vi "Get SmartCard Variable Names.vi"(8 "error in":errorcluster, 11 "Dataset Name":string) -> (0 "error out":errorcluster, 3 "Variable Names":string[](array[string]))   [LabVIEW 2015, in "Support VIs.lvlib"]
uses:
  QMH_Topside/Support VIs/Support VIs.lvlib
panel:
  out "name":string
  out "text":string
  out "stripped path":path
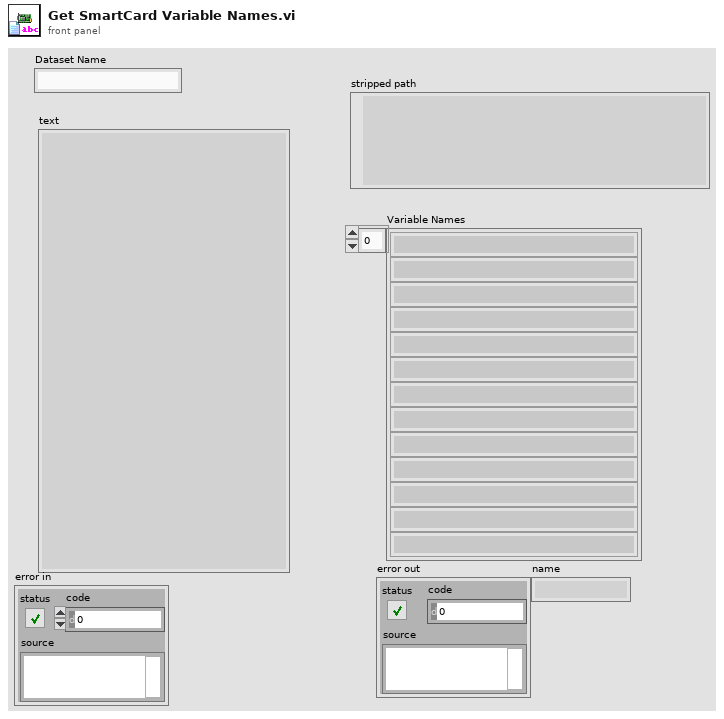
[diagram p1: front panel]
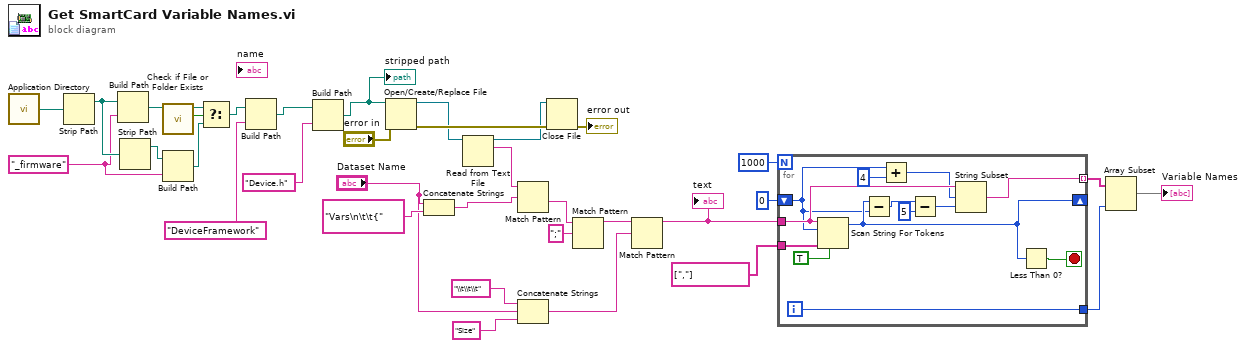
[diagram p0: block diagram]
diagram:
  w2 = "_firmware" ("name or relative path")
  n1 = call <vilib>:"Application Directory.vi"() -> ("Application Directory"=w35:path)
  n2 = Strip Path(path=w35) -> (stripped path=w4:path)  [unwired: 1 out]
  n3 = Build Path(base path=w4, name or relative path=w2) -> (appended path=w5:path)
  n4 = Strip Path(path=w4) -> (stripped path=w3:path)  [unwired: 1 out]
  n5 = call <vilib>:"Check if File or Folder Exists.vi"("path"=w5) -> ("file or folder exists?"=w8:bool, "dup path"=w7:path)  [unwired: 8 in, 1 out]
  n6 = Build Path(base path=w3, name or relative path=w2) -> (appended path=w1:path)
  n7 = Select(t=w7, s=w8, f=w1) -> (s? t:f=w6:path)
  n8 = Build Path(base path=w6, name or relative path="DeviceFramework") -> (appended path=w11:path)
  n9 = Build Path(base path=w11, name or relative path="Device.h") -> (appended path=w33:path)
  "stripped path" <- w33
  n10 = Open/Create/Replace File(file path (use dialog)=w33, error in="error in") -> (refnum out=w31:refnum<file>, error out=w32:errorcluster)  [unwired: 4 in, 1 out]
  n11 = Concatenate Strings("Dataset Name", "Vars\n\t\t{" ("regular expression")) -> (w20:string)
  n12 = Read from Text File(file (use dialog)=w31) -> (refnum out=w30:refnum<file>, text=w29:string)  [unwired: 3 in, 2 out]
  n13 = Match Pattern(string=w29, regular expression=w20) -> (after substring=w28:string)  [unwired: 1 in, 3 out]
  n14 = Concatenate Strings("\\t\\t\\t" ("string"), "Dataset Name", "Size" ("string")) -> (w16:string)
  n15 = Close File(refnum=w30, error in=w32) -> (error out=→"error out":errorcluster)  [unwired: 1 out]
  n16 = Match Pattern(string=w28, regular expression=";") -> (before substring=w25:string)  [unwired: 1 in, 3 out]
  n17 = Match Pattern(string=w25, regular expression=w16) -> (before substring=w24:string)  [unwired: 1 in, 3 out]
  "text" <- w24
  n18 = for {
    N: 1000 -> [_]
    tunnel: string[] [","] ("delimiters (\\s,\\t,\\r,\\n)") -> [w48]
    shift-right: [w41] -> _
    shift-left: 0 ("offset past token") -> [w40]
    tunnel: w24 -> [w45]
    tunnel: [w37] -> w15 mode=indexing
    tunnel: [w36] -> w13
    i -> [w36]
    stop <- w46 stop-if-true
    n19 = Scan String For Tokens(4:TRUE ("use cached delim/oper data? (F)"), 6:w48, 8:w40, 9:w45) -> (2:w41:i32)  [unwired: 2 in, 3 out]
    n20 = Subtract(x=w41, y=w40) -> (x-y=w43:i32)
    n21 = Add(x=w40, y=4) -> (x+y=w38:i32)
    n22 = Subtract(x=w43, y=5) -> (x-y=w44:i32)
    n23 = String Subset(string=w45, offset (0)=w38, length (rest)=w44) -> (substring=w37:string)
    n24 = Less Than 0?(x=w41) -> (x < 0?=w46:bool)
  }
  n25 = Array Subset(array=w15, length=w13) -> (→"Variable Names":string[])  [unwired: 1 in]
